vi "Determine Warning State Machine.vi"(6 "Max Wind Speed":dbl, 7 "Current Wind Speed":dbl, 8 "error in (no error)":errorcluster, 9 "Min Temp":dbl, 10 "Max Temp":dbl, 11 "Current Temp":dbl) -> (0 "error out":errorcluster, 1 "Warning?":bool, 2 "Warning Text":string)   [LabVIEW 2010]
doc: "This VI is a scalable, maintainable, and readable version of inherited code used as an exercise in LabVIEW Core II."
uses:
  Det Warnings.ctl
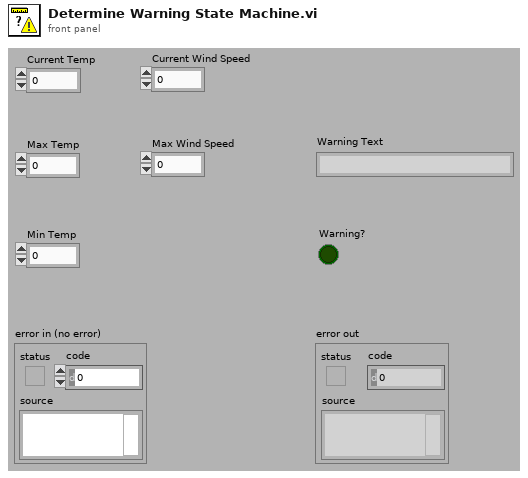
[diagram p1: front panel]
types:
  T1 = typedef "Det Warnings.ctl" = enum16{"Heatstroke", "Freeze", "High Wind", "Generate Warning"}
  T2 = cluster{"Current Temp":dbl, "Max Temp":dbl, "Min Temp":dbl, "Current Wind Speed":dbl, "Max Wind Speed":dbl}
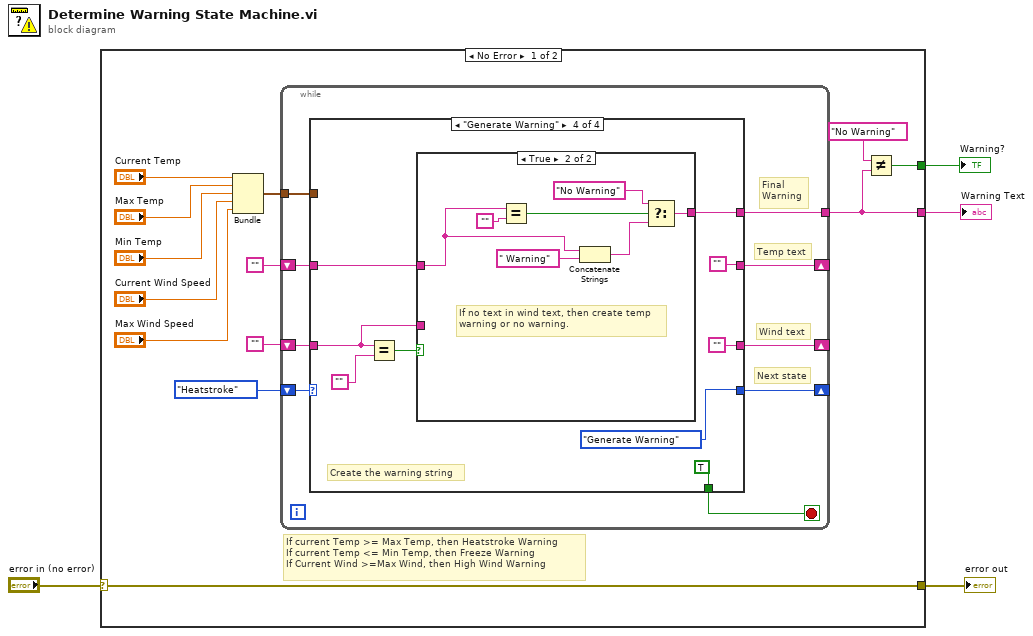
[diagram p0: block diagram]
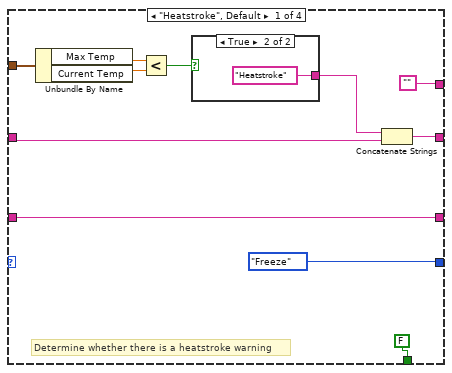
[diagram p2: hidden frame]
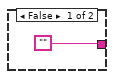
[diagram p3: hidden frame]
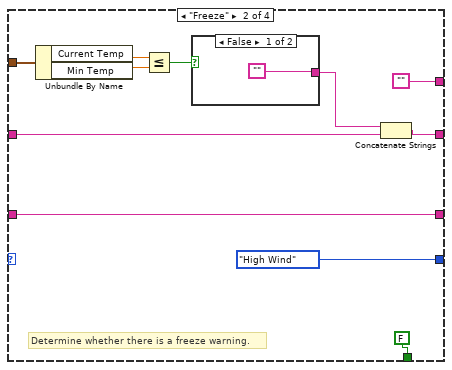
[diagram p4: hidden frame]
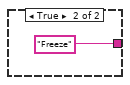
[diagram p5: hidden frame]
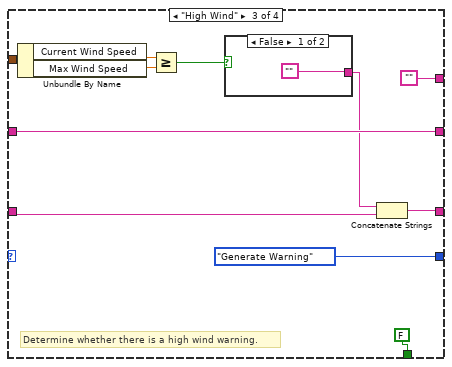
[diagram p6: hidden frame]
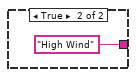
[diagram p7: hidden frame]
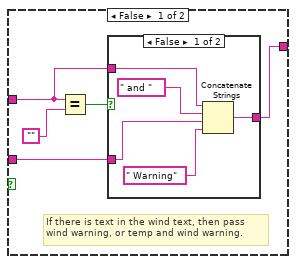
[diagram p8: hidden frame]
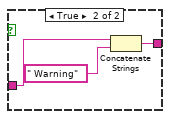
[diagram p9: hidden frame]
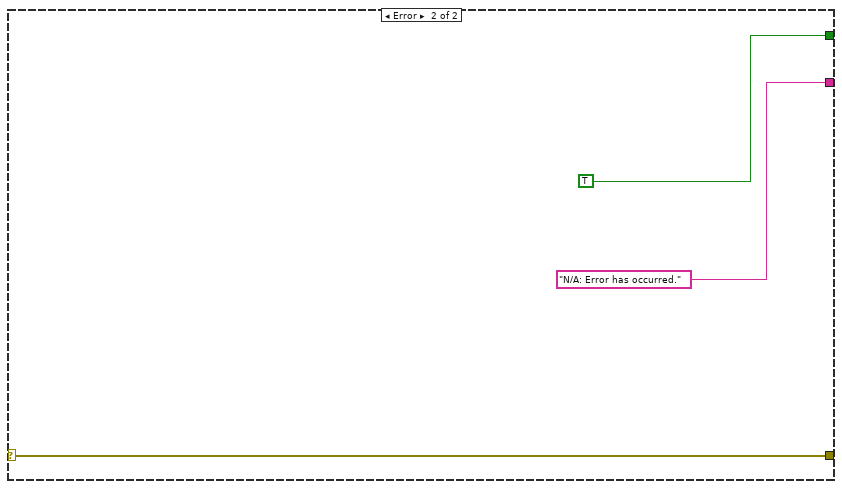
[diagram p10: hidden frame]
diagram:
  n1 = case shown="No Error" "error in (no error)" {
    selector: "error in (no error)" -> [w16 w97]
    tunnel: [w16 w97] -> w3
    tunnel: [w17 TRUE] -> w2
    tunnel: [w6 "N/A: Error has occurred." ("f")] -> w1
    frame No Error {
      # "If current Temp >= Max Temp, then Heatstroke Warning\nIf current Temp <= Min Temp, then Freeze Warning\nIf Current Wind >=Max Wind, then High Wind Warning"
      n2 = Bundle("Current Temp"="Current Temp", "Max Temp"="Max Temp", "Min Temp"="Min Temp", "Current Wind Speed"="Current Wind Speed", "Max Wind Speed"="Max Wind Speed") -> (w9:T2)  [unwired: 1 in]
      n3 = while {
        tunnel: w9 -> [w23]
        shift-right: [w22] -> _
        shift-left: Det_Warnings."Heatstroke" ("Enum") -> [w26]
        shift-right: [w25] -> _
        shift-left: "" -> [w21]
        shift-right: [w24] -> _
        shift-left: "" -> [w20]
        tunnel: [w19] -> w6
        stop <- w18 stop-if-true
        # "Final\nWarning"
        # "Next state"
        # "Wind text"
        # "Temp text"
        n4 = case shown="\"Generate Warning\"" w26 {
          tunnel: [w29 w45 w57 ""] -> w24
          tunnel: [w32 w44 w58 ""] -> w25
          tunnel: w23 -> [w36 w50 w63 _]
          tunnel: [Det_Warnings."Freeze" ("Enum") Det_Warnings."High Wind" ("Enum") Det_Warnings."Generate Warning" ("Enum") Det_Warnings."Generate Warning" ("Enum")] -> w22
          tunnel: w21 -> [w31 w42 w58 w74]
          tunnel: w20 -> [w29 w45 w55 w71]
          tunnel: ["" "" "" w70] -> w19
          tunnel: [FALSE FALSE FALSE TRUE] -> w18
          frame "Heatstroke", Default {
            # "Determine whether there is a heatstroke warning"
            n5 = Unbundle By Name(w36) -> ("Max Temp"=w35:dbl, "Current Temp"=w34:dbl)
            n6 = Less?(x=w35, y=w34) -> (x < y?=w37:bool)
            n7 = case shown="True" w37 {
              tunnel: ["" "Heatstroke"] -> w30
              frame False {
              }
              frame True {
              }
            }
            n8 = Concatenate Strings(w30, w31) -> (w32:string)
          }
          frame "Freeze" {
            # "Determine whether there is a freeze warning."
            n9 = Unbundle By Name(w50) -> ("Current Temp"=w48:dbl, "Min Temp"=w47:dbl)
            n10 = Less Or Equal?(x=w48, y=w47) -> (x <= y?=w49:bool)
            n11 = case shown="False" w49 {
              tunnel: ["" "Freeze"] -> w43
              frame False {
              }
              frame True {
              }
            }
            n12 = Concatenate Strings(w43, w42) -> (w44:string)
          }
          frame "High Wind" {
            # "Determine whether there is a high wind warning."
            n13 = Unbundle By Name(w63) -> ("Current Wind Speed"=w62:dbl, "Max Wind Speed"=w61:dbl)
            n14 = Greater Or Equal?(x=w62, y=w61) -> (x >= y?=w60:bool)
            n15 = case shown="False" w60 {
              tunnel: ["" "High Wind"] -> w56
              frame False {
              }
              frame True {
              }
            }
            n16 = Concatenate Strings(w56, w55) -> (w57:string)
          }
          frame "Generate Warning" {
            # "Create the warning string"
            n17 = Equal?(x=w71, y="") -> (x = y?=w72:bool)
            n18 = case shown="True" w72 {
              tunnel: [w77 w89] -> w70
              tunnel: w74 -> [w75 w93]
              tunnel: w71 -> [w76 _]
              frame False {
                # "If there is text in the wind text, then pass\nwind warning, or temp and wind warning."
                n19 = Equal?(x=w75, y="") -> (x = y?=w78:bool)
                n20 = case shown="False" w78 {
                  tunnel: [w82 w86] -> w77
                  tunnel: w76 -> [w81 w85]
                  tunnel: w75 -> [w80 _]
                  frame False {
                    n21 = Concatenate Strings(w80, " and " ("string"), w81, " Warning" ("string")) -> (w82:string)
                  }
                  frame True {
                    n22 = Concatenate Strings(w85, " Warning" ("string")) -> (w86:string)
                  }
                }
              }
              frame True {
                # "If no text in wind text, then create temp\nwarning or no warning."
                n23 = Equal?(x=w93, y="") -> (x = y?=w92:bool)
                n24 = Concatenate Strings(w93, " Warning") -> (w88:string)
                n25 = Select(t="No Warning" ("string"), s=w92, f=w88) -> (s? t:f=w89:string)
              }
            }
          }
        }
      }
      n26 = Not Equal?(x="No Warning", y=w6) -> (x != y?=w17:bool)
    }
    frame Error {
    }
  }
  "error out" <- w3
  "Warning Text" <- w1
  "Warning?" <- w2
